vi "calculateRangeModePositions.vi"(6 "Delay between send and receive [ms]":i32=100, 8 "error in (no error)":errorcluster, 10 "calculateRangeModePositions":T1, 11 "CCD in":refnum<class "CCD.lvclass">) -> (0 "error out":errorcluster, 2 "Positions":dbl[](array[numeric]), 3 "CCD out":refnum<class "CCD.lvclass">, 4 "results-JSON string":string)   [LabVIEW 2023, in "horiba.lvlib" / "CCD.lvclass"]
doc: "tarts an acquisition that has been set up according to the previously defined acquisition parameters.\n\nNote: To specify the acquisition parameters please see ccd_setROI and ccd_setXAxisConversionType. If there are no acquisition parameters specified at the time of acquisition it may result in no data being generated."
uses:
  CCD.lvclass
  20f7d3bd-08ac-4524-9bed-df36c1da25a0.vi
  cab240a6-cbf4-4e2c-ab79-96d9c1b88265.vi
  6968c003-a3a8-4fe6-bd53-13ad12dc6eda.vi
  d8999305-94e7-4d24-b768-1afaedf83813.vi
  4fd64012-a7af-4048-b972-7cd663129ff9.vi
  <vilib>/JDP Science/JSONtext/Variant to JSON Text.vi
  <vilib>/JDP Science/JSONtext/Set Item.vi
  <vilib>/JDP Science/JSONtext/LVClass Serializer/JSONtext LVClass Serializer.lvclass
  CCD.lvclass/CCD.ctl
  GenericDevice/GenericDevice.lvclass
  <vilib>/JDP Science/JSONtext/JSONtext.lvlib
panel:
  # "Connector Pane"
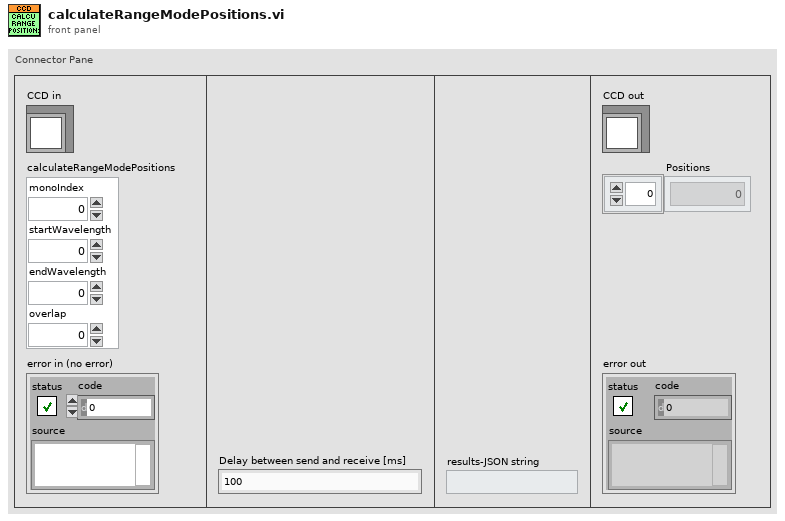
[diagram p1: front panel]
types:
  T1 = cluster{"monoIndex":i32, "startWavelength":dbl, "endWavelength":dbl, "overlap":dbl}
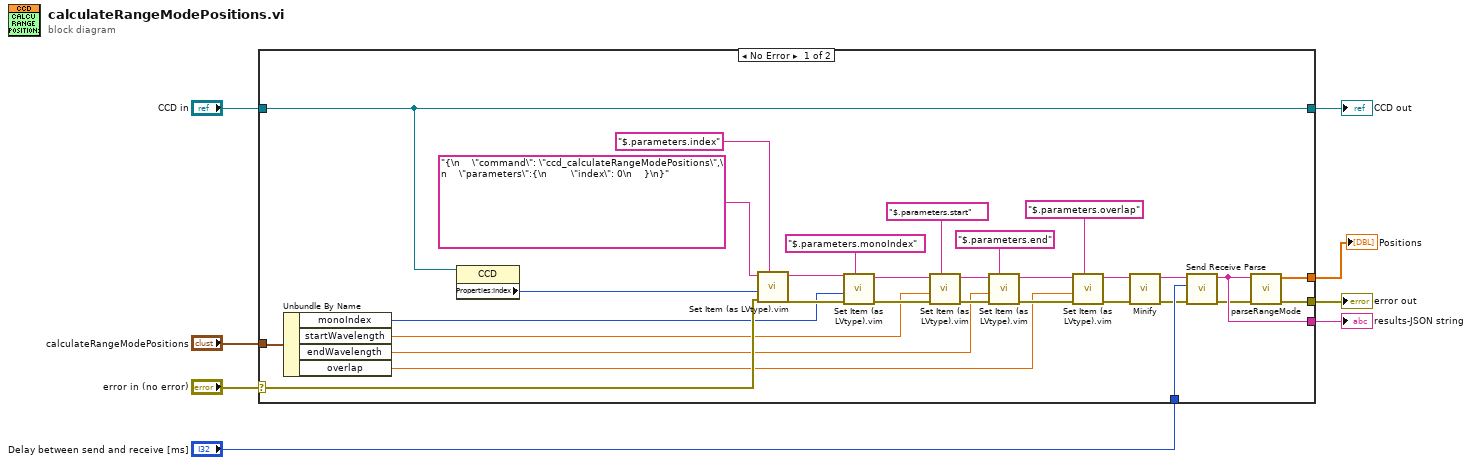
[diagram p0: block diagram]
diagram:
  n1 = case shown="No Error" "error in (no error)" {
    selector: "error in (no error)" -> [w35 w41]
    tunnel: [w13 w41] -> w7
    tunnel: [w37 w40] -> w5
    tunnel: "CCD in" -> [w37 w40]
    tunnel: [w15 _] -> w4
    tunnel: "Delay between send and receive [ms]" -> [w30 _]
    tunnel: "calculateRangeModePositions" -> [w29 _]
    tunnel: [w9 _] -> w1
    frame No Error {
      n2 = Unbundle By Name(w29) -> ("monoIndex"=w19:i32, "startWavelength"=w18:dbl, "endWavelength"=w17:dbl, "overlap"=w16:dbl)
      n3 = property class="CCD"(reference=w37) -> ("Properties:Index"=w36:i32)  [unwired: 1 in, 2 out]
      n4 = call "Set Item (as LVtype).vim"("$Path or Item Name"="$.parameters.index", "error in (no error)"=w35, "Anything"=w36, "JSON"="{\n    \"command\": \"ccd_calculateRangeModePositions\",\n    \"parameters\":{\n        \"index\": 0\n    }\n}") -> ("error out"=w33:errorcluster, "<JSON>"=w31:string)  [unwired: 4 in, 1 out]
      n5 = call "Set Item (as LVtype).vim"("$Path or Item Name"="$.parameters.monoIndex", "error in (no error)"=w33, "Anything"=w19, "JSON"=w31) -> ("error out"=w32:errorcluster, "<JSON>"=w27:string)  [unwired: 4 in, 1 out]
      n6 = call "Set Item (as LVtype).vim"("$Path or Item Name"="$.parameters.start", "error in (no error)"=w32, "Anything"=w18, "JSON"=w27) -> ("error out"=w28:errorcluster, "<JSON>"=w24:string)  [unwired: 4 in, 1 out]
      n7 = call "Set Item (as LVtype).vim"("$Path or Item Name"="$.parameters.end", "error in (no error)"=w28, "Anything"=w17, "JSON"=w24) -> ("error out"=w25:errorcluster, "<JSON>"=w21:string)  [unwired: 4 in, 1 out]
      n8 = call "Set Item (as LVtype).vim"("$Path or Item Name"="$.parameters.overlap", "error in (no error)"=w25, "Anything"=w16, "JSON"=w21) -> ("error out"=w22:errorcluster, "<JSON>"=w11:string)  [unwired: 4 in, 1 out]
      n9 = call <vilib>:"Minify.vi"("error in (no error)"=w22, "JSON"=w11) -> ("error out"=w12:errorcluster, "<JSON>"=w10:string)  [unwired: 7 in, 1 out]
      n10 = call "Send Receive Parse.vi"("error in"=w12, "Delay between send and receive [ms]"=w30, "<JSON>"=w10) -> ("error out"=w14:errorcluster, "results-JSON string"=w15:string)  [unwired: 6 in, 1 out]
      n11 = call "parseRangeMode.vi"("error in (no error)"=w14, "String"=w15) -> ("error out"=w13:errorcluster, "Data"=w9:dbl[])  [unwired: 8 in]
    }
    frame Error {
    }
  }
  "error out" <- w7
  "CCD out" <- w5
  "results-JSON string" <- w4
  "Positions" <- w1
